vi "Main.vi"() -> ()   [LabVIEW 2019]
panel:
  in  "stop":bool
  out "Numeric 2":dbl
  in  "Numeric":dbl
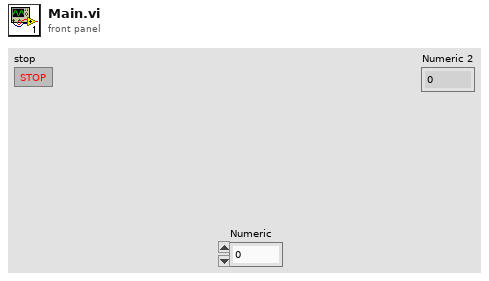
[diagram p1: front panel]
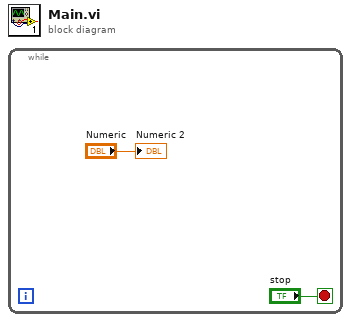
[diagram p0: block diagram]
diagram:
  n1 = while {
    stop <- "stop" stop-if-true
    "Numeric 2" <- "Numeric"
  }
